vi "T15.vi"(2 "Parametry Ziemi":T1={"a - półoś duża"=6378137.0, "b - półoś mała"=6356752.3141999999998} {"b - półoś mała" format="%_20f"; "a - półoś duża" format="%_20g"}, 3 "fi'":ext) -> (7 "T15":ext)   [LabVIEW 2015, in "Biblioteka moduł map v3.lvlib" / "Konwersja wsp.lvlib" / "UTM.lvlib" / "Konwersja z UTM na wsp geograficzne.lvlib"]
uses:
  Konwersja z UTM na wsp geograficzne.lvlib
  UTM.lvlib
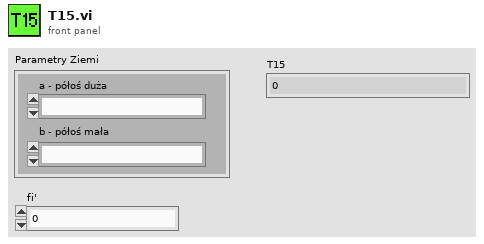
[diagram p1: front panel]
types:
  T1 = cluster{"a - półoś duża":ext, "b - półoś mała":ext}
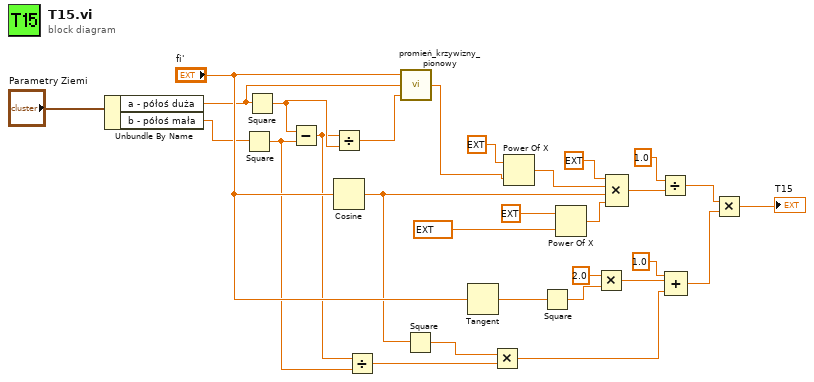
[diagram p0: block diagram]
diagram:
  n1 = Unbundle By Name("Parametry Ziemi") -> ("a - półoś duża"=w2:ext, "b - półoś mała"=w1:ext)
  n2 = Square(x=w1) -> (x^2=w5:ext)
  n3 = Square(x=w2) -> (x^2=w29:ext)
  n4 = Subtract(x=w29, y=w5) -> (x-y=w6:ext)
  n5 = Divide(x=w6, y=w29) -> (x/y=w28:ext)
  n6 = Cosine(x="fi'") -> (cos(x)=w9:ext)
  n7 = Divide(x=w6, y=w5) -> (x/y=w4:ext)
  n8 = call "promień_krzywizny_pionowy.vi"("e^2"=w28, "a"=w2, "fi[rad]"="fi'") -> ("Promien krzywizny równoleżnika"=w25:dbl)  [unwired: 2 in]
  n9 = Square(x=w9) -> (x^2=w8:ext)
  n10 = Tangent(1:"fi'") -> (0:w10:ext)
  n11 = Multiply(x=w8, y=w4) -> (x*y=w7:ext)
  n12 = Power Of X(1:w25, 2:ext 3.0 ("y")) -> (0:w23:ext)
  n13 = Square(x=w10) -> (x^2=w11:ext)
  n14 = Power Of X(1:ext 0.9996 ("k0"), 2:ext 3.0 ("y")) -> (0:w19:ext)
  n15 = Multiply(x=2.0, y=w11) -> (x*y=w13:ext)
  n16 = Compound Arithmetic op=MULTIPLY(ext 6.0 ("value"), w23, w9, w19) -> (w26:ext)
  n17 = Divide(x=1.0, y=w26) -> (x/y=w18:ext)
  n18 = Compound Arithmetic op=ADD(1.0 ("value"), w13, w7) -> (w17:ext)
  n19 = Multiply(x=w18, y=w17) -> (x*y=→"T15":ext)
